vi "test_libssh2_channel_window_write_ex.vi"() -> ()   [LabVIEW 2013, in "libssh2_integration_tests.lvlib"]
uses:
  libssh2_integration_tests.lvlib
  <vilib>/addons/_JKI Toolkits/Caraya/classes/Test/Test.lvclass
  libssh2/libssh2.lvlib
  <vilib>/addons/_JKI Toolkits/Caraya/classes/Assert/Assert.lvclass
panel:
  out "error out":errorcluster
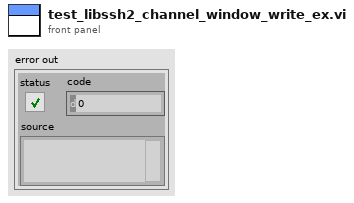
[diagram p1: front panel]
types:
  T1 = typedef "libssh2.lvlib/Session Refnum.ctl" = refnum<k1>
  T2 = typedef "libssh2.lvlib/Channel Refnum.ctl" = refnum<k1>
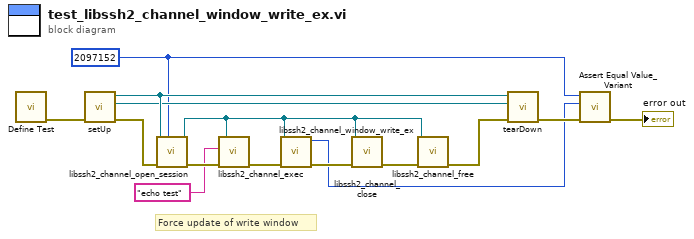
[diagram p0: block diagram]
diagram:
  w5 = u32 2097152 ("window_size (2 MiB)")
  # "Force update of write window"
  n1 = call <vilib>:"Define Test.vi"() -> ("error out"=w14:errorcluster)  [unwired: 10 in, 1 out]
  n2 = call "setUp.vi"("error in (no error)"=w14) -> ("error out"=w9:errorcluster, "connection ID"=w11:refnum<k5>, "session"=w12:T1)  [unwired: 8 in]
  n3 = call "libssh2_channel_open_session.vi"("window_size (2 MiB)"=w5, "error in (no error)"=w9, "session"=w12) -> ("error out"=w6:errorcluster, "channel"=w3:T2)  [unwired: 7 in]
  n4 = call "libssh2_channel_exec.vi"("error in (no error)"=w6, "command"="echo test", "channel"=w3) -> ("error out"=w4:errorcluster)  [unwired: 8 in]
  n5 = call "libssh2_channel_window_write_ex.vi"("error in (no error)"=w4, "channel"=w3) -> ("error out"=w7:errorcluster, "remaining write window"=w1:u32)  [unwired: 7 in, 1 out]
  n6 = call "libssh2_channel_close.vi"("error in (no error)"=w7, "channel"=w3) -> ("error out"=w10:errorcluster)  [unwired: 9 in]
  n7 = call "libssh2_channel_free.vi"("error in (no error)"=w10, "channel"=w3) -> ("error out"=w8:errorcluster)  [unwired: 9 in]
  n8 = call "tearDown.vi"("error in (no error)"=w8, "connection ID"=w11, "session"=w12) -> ("error out"=w13:errorcluster)  [unwired: 8 in]
  n9 = call <vilib>:"Assert Equal Value_Variant.vi"("error in (no error)"=w13, "Y"=w1, "X"=w5) -> ("error out"=→"error out":errorcluster)  [unwired: 7 in, 1 out]
